vi "IMAQdx Open Camera.vi"(7 "Camera Control Mode":T2, 8 "error in":errorcluster, 11 "Session In":T1) -> (0 "error out":errorcluster, 3 "Session Out":T1)   [LabVIEW 2020, in "NI_Vision_Acquisition_Software.lvlib"]
doc: "Opens a camera, queries the camera for its capabilities, loads a camera configuration file, and creates a unique reference to the camera. Use the IMAQdx Close Camera VI when you are finished with the reference."
uses:
  NI_Vision_Acquisition_Software.lvlib
  IMAQdx.ctl
  IMAQdx Camera Control Mode.ctl
  niimaqdx.dll
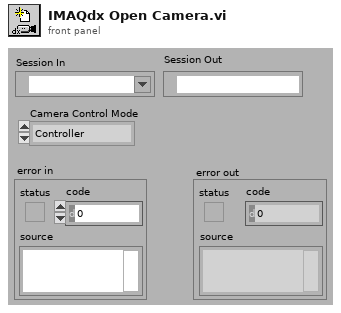
[diagram p1: front panel]
types:
  T1 = typedef "IMAQdx.ctl" = refnum<k21>
  T2 = typedef "NI_Vision_Acquisition_Software.lvlib/IMAQdx Camera Control Mode.ctl" = enum32{"Controller", "Listener"}
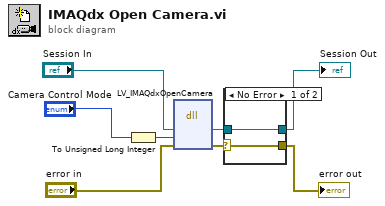
[diagram p0: block diagram]
diagram:
  n1 = To Unsigned Long Integer(number="Camera Control Mode") -> (unsigned 32bit integer=w7:u32)
  n2 = dll-call lib="niimaqdx.dll" fn="LV_IMAQdxOpenCamera"("Session In"="Session In", "mode"=w7, "error in"="error in") -> ("Session In"=w2:T1, "error in"=w4:errorcluster)  [unwired: 5 in, 2 out]
  n3 = case shown="No Error" w4 {
    selector: w4 -> [w10 w11]
    tunnel: [w10 w11] -> w3
    tunnel: w2 -> [w9 _]
    tunnel: [w9 _] -> w1
    frame No Error {
    }
    frame Error {
    }
  }
  "Session Out" <- w1
  "error out" <- w3
